vi "counter-delta.vi"(8 "error in (no error)":errorcluster, 11 "command line":string) -> (0 "error out":errorcluster, 2 "standard error":string, 3 "Numeric":dbl)   [LabVIEW 2023]
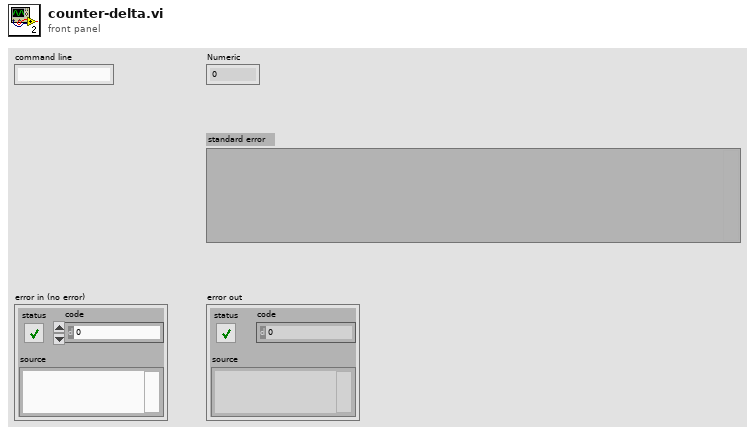
[diagram p1: front panel]
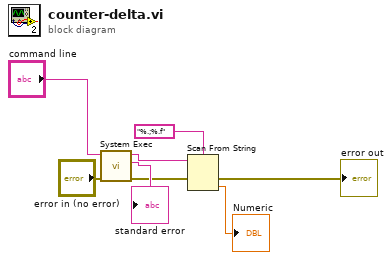
[diagram p0: block diagram]
diagram:
  n1 = call <vilib>:"System Exec.vi"("error in (no error)"="error in (no error)", "command line"="command line") -> ("error out"=w4:errorcluster, "standard error"=→"standard error":string, "standard output"=w2:string)  [unwired: 6 in, 1 out]
  n2 = Scan From String(format string="%.;%.f", input string=w2, error in=w4) -> (error out=→"error out":errorcluster, output 1=→"Numeric":dbl)  [unwired: 2 in, 2 out]
